vi "demande_achat_et_gestion_delais.vi"() -> ()   [LabVIEW 2021]
uses:
  <vilib>/numeric/Random Number (Range) U64.vi
  <vilib>/numeric/sub_Random U32.vi
panel:
  out "Livraison à temps":bool
  out "delai attente":dbl
  in  "Delai de livraison client":dbl
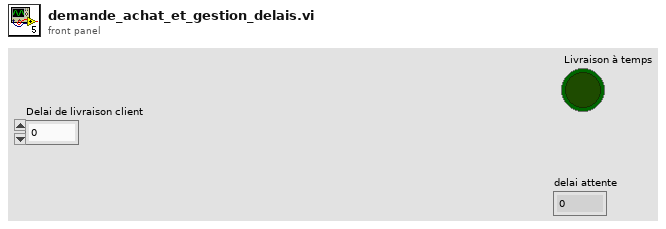
[diagram p1: front panel]
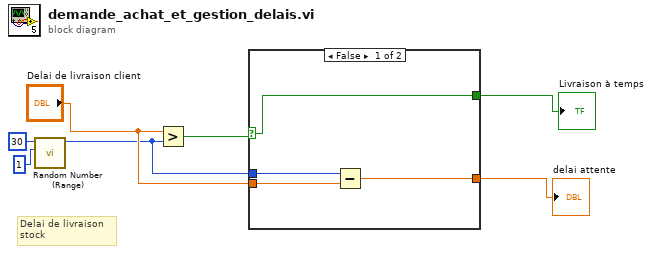
[diagram p0: block diagram]
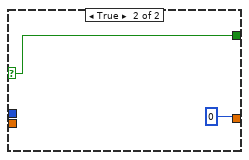
[diagram p2: hidden frame]
diagram:
  # "Delai de livraison stock"
  n1 = call-poly <vilib>:"Random Number (Range).vi"("lower bound (0)"=u64 1, "upper bound (100)"=u64 30) -> ("number"=w1:u64)  [unwired: 9 in]
  n2 = Greater?(x="Delai de livraison client", y=w1) -> (0:w5:bool)
  n3 = case shown="False" w5 {
    selector: w5 -> [w11 w13]
    tunnel: [w11 w13] -> w4
    tunnel: [w8 0] -> w3
    tunnel: "Delai de livraison client" -> [w9 _]
    tunnel: w1 -> [w10 _]
    frame False {
      n4 = Subtract(x=w10, y=w9) -> (x-y=w8:dbl)
    }
    frame True {
    }
  }
  "delai attente" <- w3
  "Livraison à temps" <- w4
